vi "Parse Fit.vi"(8 "Error In":errorcluster, 11 "File Path":path) -> (0 "Error Out":errorcluster)   [LabVIEW 2016]
panel:
  out "Width":dbl[](array[numeric])
  out "Amplitude":dbl[](array[numeric])
  out "F":dbl[](array[numeric])
  out "F names":string[](array[string])
  out "Amplitude names":string[](array[string])
  out "Width names":string[](array[string])
  out "Array - String":string[](array[string])
  out "group name out":string
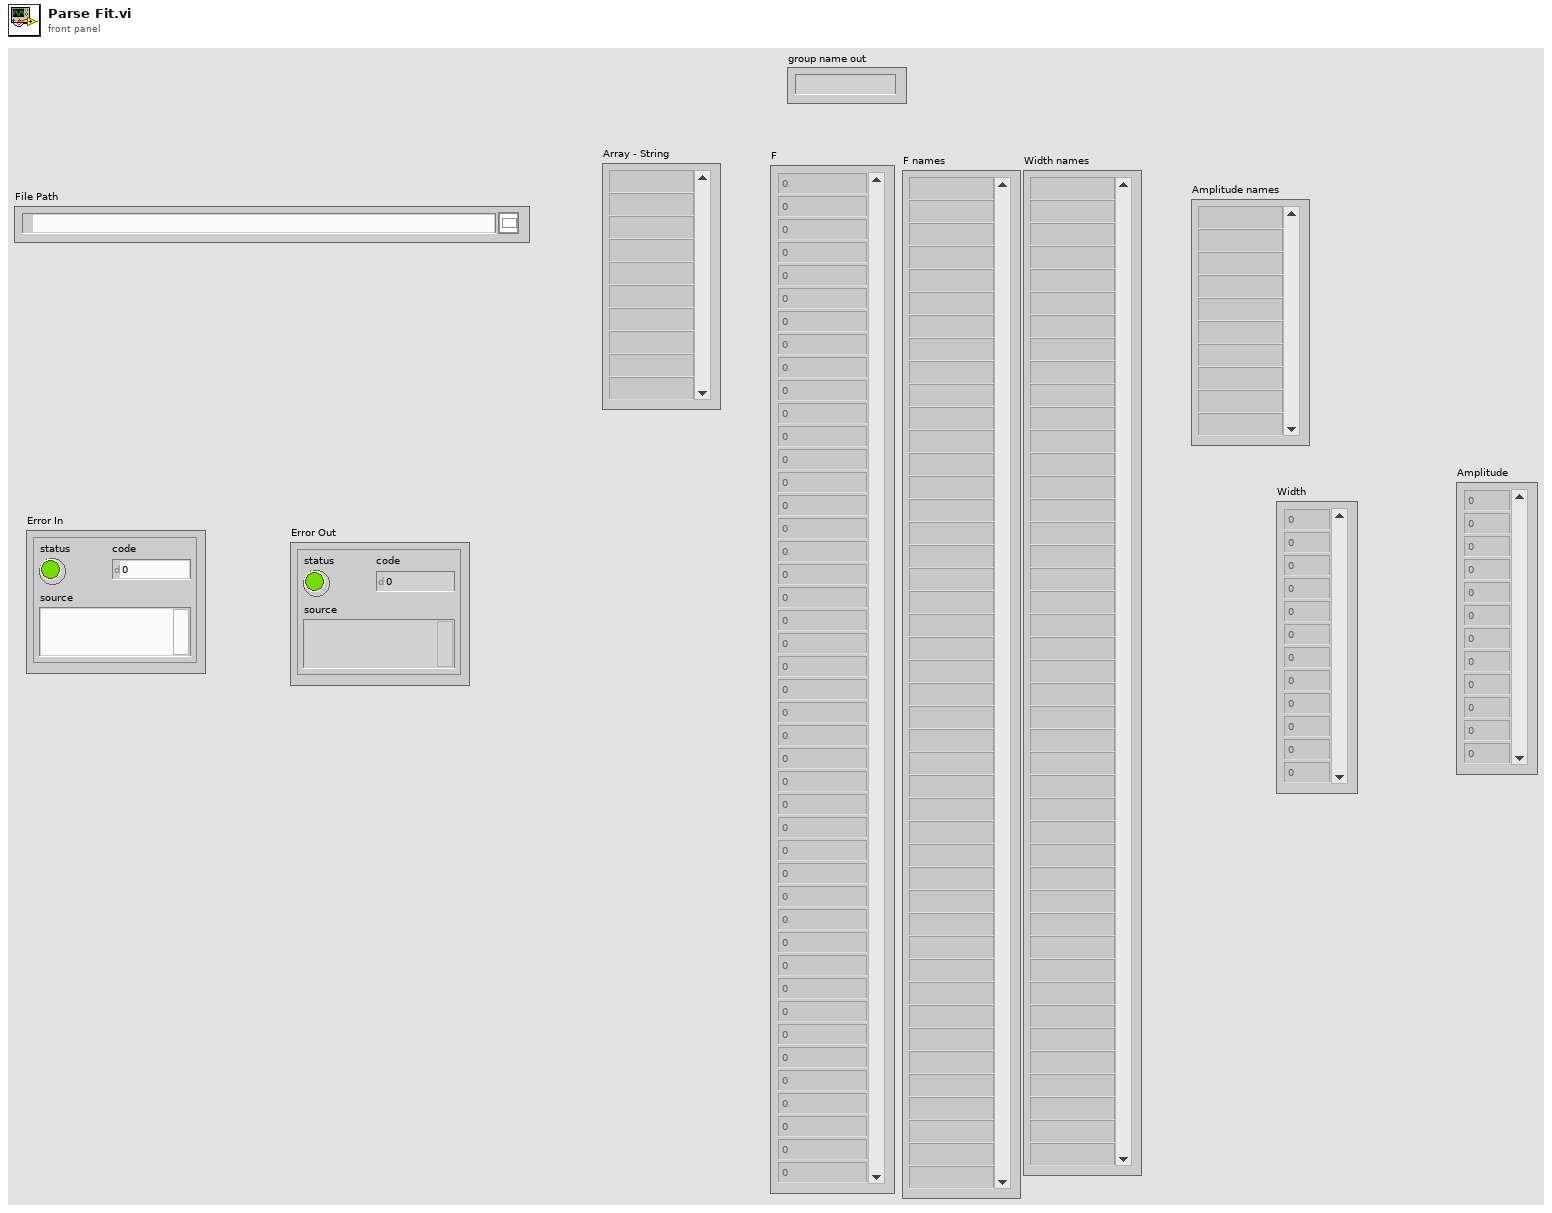
[diagram p1: front panel]
types:
  T1 = enum16{"open", "open or create", "create or replace", "create", "open (read-only)"}
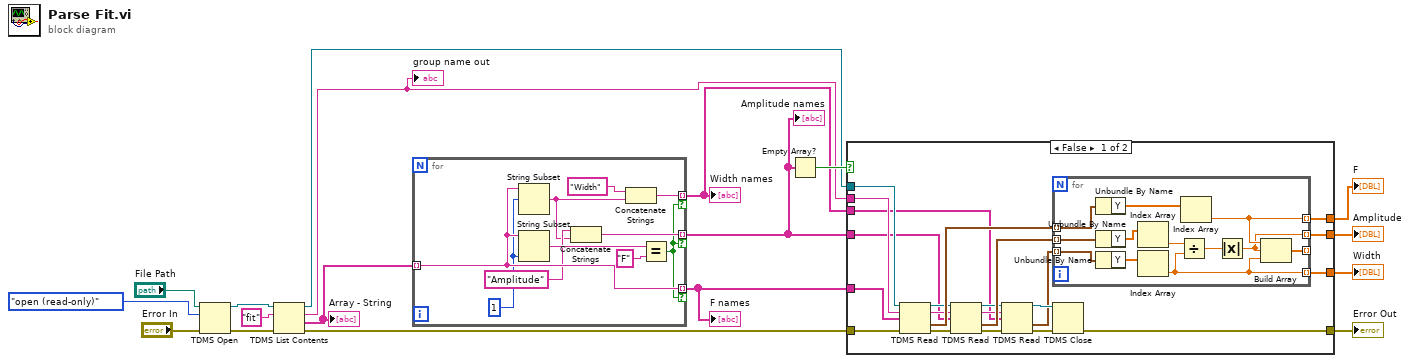
[diagram p0: block diagram]
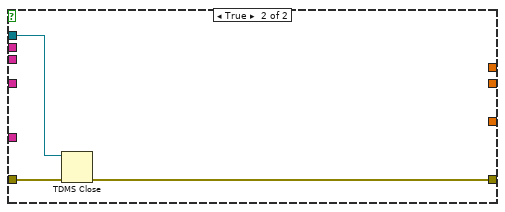
[diagram p2: hidden frame]
diagram:
  n1 = TDMS Open(8:"Error In", 10:T1."open (read-only)" ("operation (0:open)"), 11:"File Path") -> (0:w15:errorcluster, 3:w13:refnum<k34>)  [unwired: 4 in]
  n2 = TDMS List Contents(4:w15, 6:"fit" ("group name"), 7:w13) -> (0:w9:errorcluster, 1:w12:string[], 2:w7:string, 3:w10:refnum<k34>)
  "group name out" <- w7
  "Array - String" <- w12
  n3 = for {
    tunnel: w12 -> [w26] mode=indexing
    tunnel: [w26] -> w5 mode=indexing if=w19
    tunnel: [w23] -> w6 mode=indexing if=w19
    tunnel: [w20] -> w4 mode=indexing if=w19
    w25 = 1 ("length (rest)")
    n4 = String Subset(string=w26, offset (0)=w25) -> (substring=w21:string)  [unwired: 1 in]
    n5 = String Subset(string=w26, length (rest)=w25) -> (substring=w28:string)  [unwired: 1 in]
    n6 = Concatenate Strings("Amplitude" ("y"), w21) -> (w23:string)
    n7 = Concatenate Strings("Width" ("y"), w21) -> (w20:string)
    n8 = Equal?(x=w28, y="F") -> (x = y?=w19:bool)
  }
  "Width names" <- w4
  "Amplitude names" <- w6
  "F names" <- w5
  n9 = Empty Array?(array=w6) -> (empty?=w11:bool)
  n10 = case shown="False" w11 {
    tunnel: [w38 w64] -> w8
    tunnel: w10 -> [w37 w62]
    tunnel: w9 -> [w36 w63]
    tunnel: w7 -> [w35 _]
    tunnel: w6 -> [w34 _]
    tunnel: w5 -> [w33 _]
    tunnel: w4 -> [w32 _]
    tunnel: [w31 _] -> w3
    tunnel: [w30 _] -> w2
    tunnel: [w29 _] -> w1
    frame False {
      n11 = TDMS Read(0:w37, 5:w35, 7:w33, 11:w36) -> (4:w48:refnum<k34>, 6:w47:string, 10:w49:waveform(dbl)[], 15:w46:errorcluster)  [unwired: 4 in, 2 out]
      n12 = TDMS Read(0:w48, 5:w47, 7:w34, 11:w46) -> (4:w44:refnum<k34>, 6:w40:string, 10:w45:waveform(dbl)[], 15:w43:errorcluster)  [unwired: 4 in, 2 out]
      n13 = TDMS Read(0:w44, 5:w40, 7:w32, 11:w43) -> (4:w41:refnum<k34>, 10:w39:waveform(dbl)[], 15:w42:errorcluster)  [unwired: 4 in, 3 out]
      n14 = for {
        tunnel: w49 -> [w61] mode=indexing
        tunnel: [w54] -> w31 mode=indexing
        tunnel: w45 -> [w59] mode=indexing
        tunnel: [w51] -> w30 mode=indexing
        tunnel: w39 -> [w58] mode=indexing
        tunnel: [w52] -> _ mode=indexing
        tunnel: [w50] -> w29 mode=indexing
        n15 = Unbundle By Name(w61) -> ("Y"=w60:dbl[])
        n16 = Unbundle By Name(w59) -> ("Y"=w56:dbl[])
        n17 = Unbundle By Name(w58) -> ("Y"=w57:dbl[])
        n18 = Index Array(array=w56) -> (element=w53:dbl)  [unwired: 1 in]
        n19 = Index Array(array=w57) -> (element=w50:dbl)  [unwired: 1 in]
        n20 = Divide(x=w53, y=w50) -> (x/y=w55:dbl)
        n21 = Index Array(array=w60) -> (element=w54:dbl)  [unwired: 1 in]
        n22 = Absolute Value(x=w55) -> (abs(x)=w51:dbl)
        n23 = Build Array(w54, w51, w50) -> (w52:dbl[])
      }
      n24 = TDMS Close(8:w42, 11:w41) -> (0:w38:errorcluster)  [unwired: 1 out]
    }
    frame True {
      n25 = TDMS Close(8:w63, 11:w62) -> (0:w64:errorcluster)  [unwired: 1 out]
    }
  }
  "Error Out" <- w8
  "F" <- w3
  "Amplitude" <- w2
  "Width" <- w1
